vi "pm1-fpga.vi"(0 "Active4":sgl, 1 "f4 (periods/tick)":sgl format="%.5f", 2 "Active3":sgl, 3 "f3 (periods/tick)":sgl format="%.5f", 4 "Active2":sgl, 5 "f2 (periods/tick)":sgl format="%.5f", 6 "Active1":sgl, 7 "f1 (periods/tick)":sgl format="%.5f", 20 "stop":bool, 27 "volume":sgl) -> (24 "AccZ":sgl, 25 "AccY":sgl, 26 "AccX":sgl)   [LabVIEW 2015]
uses:
  <vilib>/rvi/Emulation/niFpgaGetClockAttributes.vi
  <vilib>/rvi/Emulation/niFpgaSctlEmulationGetInTimedLoop.vi
  <vilib>/rvi/Emulation/niFpgaEmulationReportErrorSimple.vi
  <vilib>/rvi/eio/common/nirviEmuTemplateMethod_errors.vi
  <vilib>/rvi/Emulation/niFpgaCriticalErrorInLSC.vi
  <vilib>/eio/EIONode/EIONode.xnode
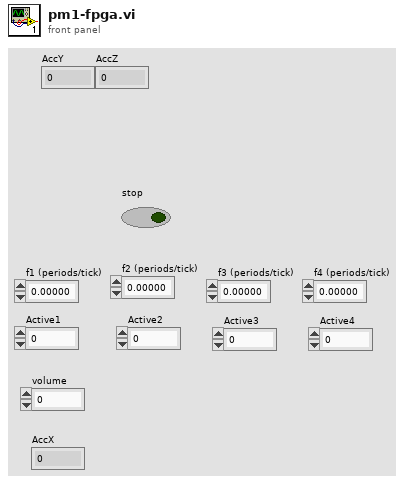
[diagram p1: front panel]
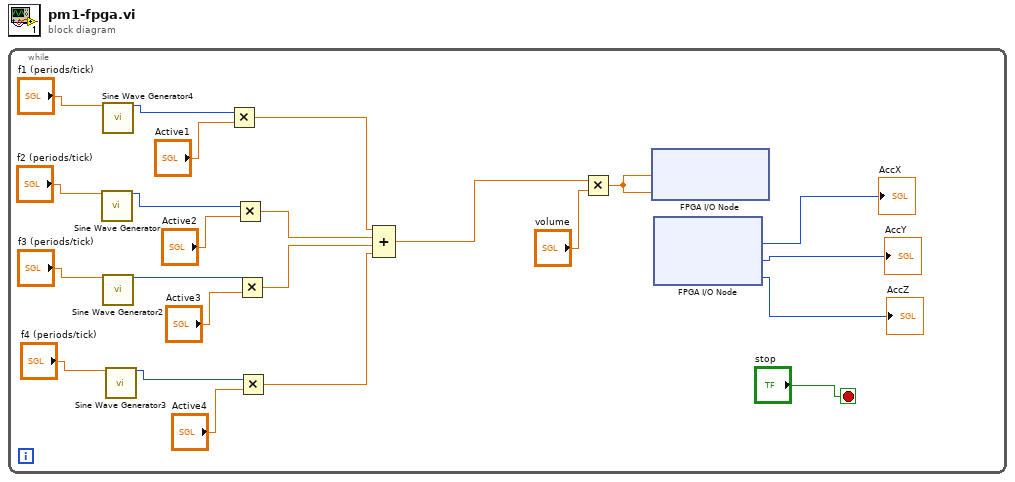
[diagram p0: block diagram]
diagram:
  n1 = while {
    stop <- "stop" stop-if-true
    n2 = call "Sine Wave Generator"("frequency (periods/tick)"="f2 (periods/tick)") -> ("sine out"=w15:i16)  [unwired: 14 in]
    n3 = call "Sine Wave Generator4"("frequency (periods/tick)"="f1 (periods/tick)") -> ("sine out"=w16:i16)  [unwired: 14 in]
    n4 = call "Sine Wave Generator2"("frequency (periods/tick)"="f3 (periods/tick)") -> ("sine out"=w14:i16)  [unwired: 14 in]
    n5 = call "Sine Wave Generator3"("frequency (periods/tick)"="f4 (periods/tick)") -> ("sine out"=w13:i16)  [unwired: 14 in]
    n6 = Multiply(x=w16, y="Active1") -> (x*y=w7:sgl)
    n7 = Multiply(x=w15, y="Active2") -> (x*y=w6:sgl)
    n8 = Multiply(x=w14, y="Active3") -> (x*y=w4:sgl)
    n9 = Multiply(x=w13, y="Active4") -> (x*y=w5:sgl)
    n10 = Compound Arithmetic op=ADD(w7, w6, w4, w5) -> (w8:sgl)
    n11 = Multiply(x=w8, y="volume") -> (x*y=w17:sgl)
    n12 = xnode "FPGA I/O Node"("AudioOut/Left"=w17, "AudioOut/Right"=w17) -> ()  [unwired: 2 in, 2 out]
    n13 = xnode "FPGA I/O Node"() -> ("AccelerationX"=→"AccX":i16, "AccelerationY"=→"AccY":i16, "AccelerationZ"=→"AccZ":i16)  [unwired: 3 in, 3 out]
  }
